vi "Calibration-NormalizeData.vi"(8 "error in (no error)":errorcluster, 11 "Calibration-RunTest in":refnum<class "Calibration-RunTest.lvclass">) -> (0 "error out":errorcluster, 3 "Calibration-RunTest out":refnum<class "Calibration-RunTest.lvclass">)   [LabVIEW 2013]
uses:
  Calibration-RunTest.lvclass
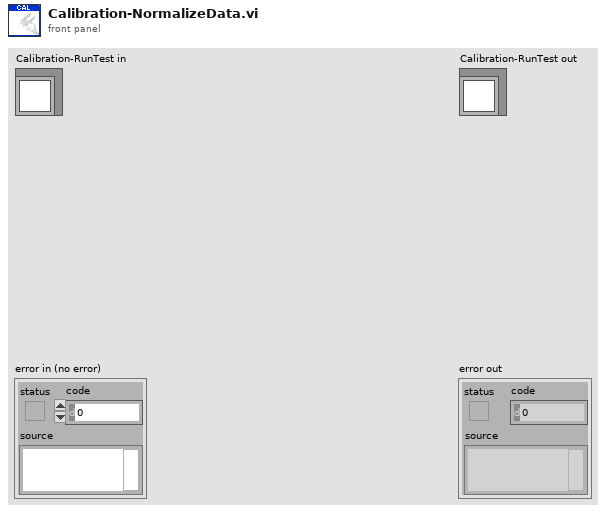
[diagram p1: front panel]
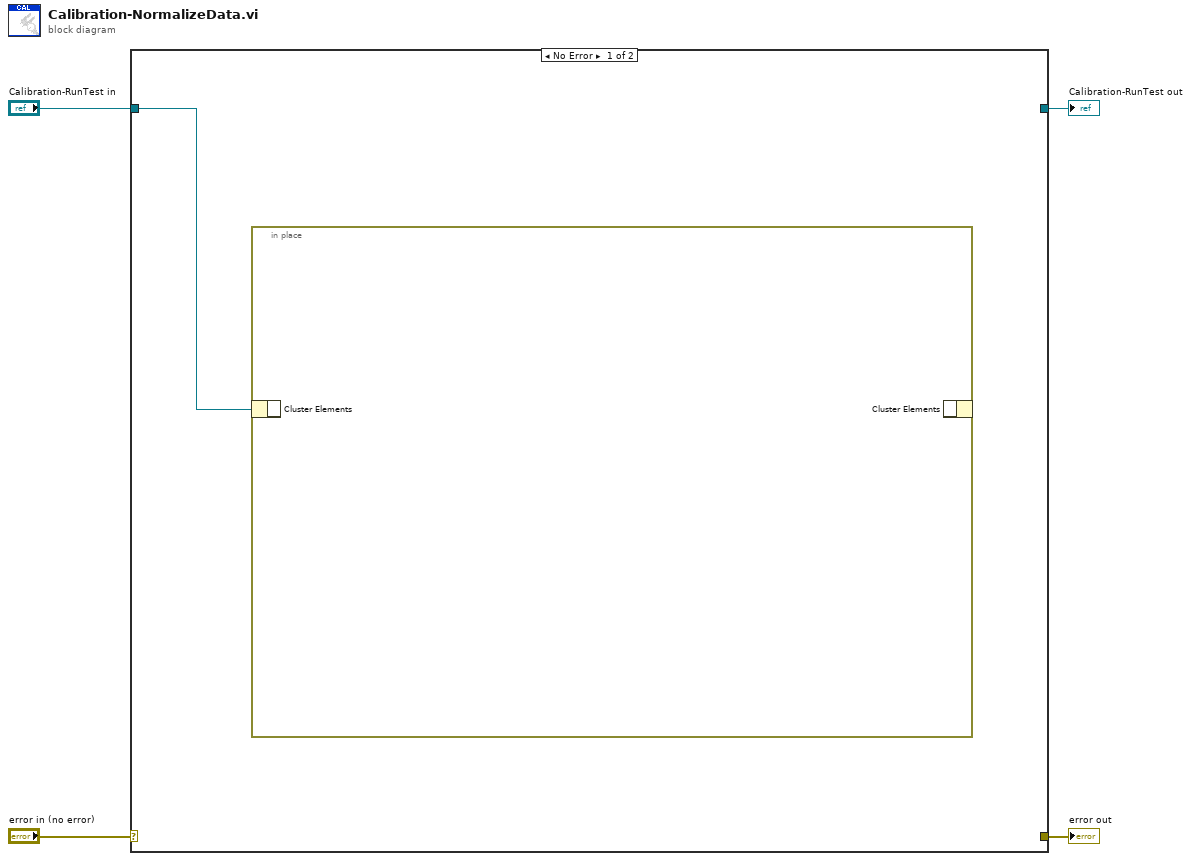
[diagram p0: block diagram]
diagram:
  n1 = case shown="No Error" "error in (no error)" {
    selector: "error in (no error)" -> [_ w7]
    tunnel: [_ w7] -> w3
    tunnel: [_ w6] -> w1
    tunnel: "Calibration-RunTest in" -> [w5 w6]
    frame No Error {
      n2 = in-place {
        n3 = in-place-cluster #1(w5) -> ()  [unwired: 1 out]
        n4 = in-place-cluster #1() -> ()  [unwired: 1 in, 1 out]
      }
    }
    frame Error {
    }
  }
  "error out" <- w3
  "Calibration-RunTest out" <- w1
